vi "Highlight failed parts(Table).vi"(8 "error in (no error)":errorcluster, 10 "Tbl Refnum":refnum<vi>, 11 "Fail array":bool[](array[boolean])) -> (0 "error out":errorcluster)   [LabVIEW 2015, in "ZenGage v3.0 UI.lvclass"]
uses:
  ZenGage v3.0 UI.lvclass
  <vilib>/Utility/miscctls.llb/LVRowAndColumnTypeDef.ctl
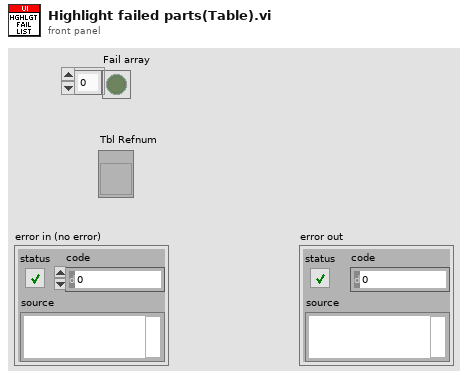
[diagram p1: front panel]
types:
  T1 = typedef "LVRowAndColumnTypeDef.ctl" = cluster{"Row":i32, "Column":i32}
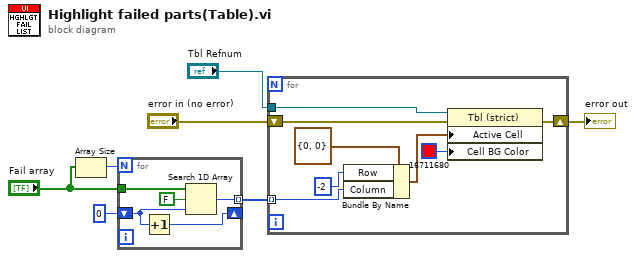
[diagram p0: block diagram]
diagram:
  n1 = Array Size(array="Fail array") -> (size(s)=w3:i32)
  n2 = for {
    N: w3 -> [_]
    tunnel: "Fail array" -> [w12]
    shift-right: [w8] -> _
    shift-left: 0 ("index of element") -> [w9]
    tunnel: [w10] -> w6 mode=indexing
    n3 = Increment(x=w9) -> (x+1=w8:i32)
    n4 = Search 1D Array(1D array=w12, element=FALSE, start index (0)=w9) -> (index of element=w10:i32)
  }
  n5 = for {
    tunnel: w6 -> [w17] mode=indexing
    shift-right: [w15] -> w4
    shift-left: "error in (no error)" -> [w16]
    tunnel: "Tbl Refnum" -> [w13]
    n6 = Bundle By Name(cluster=T1 {"Row"=0, "Column"=0} ("Active Cell:Active Cell"), "Row"=-2, "Column"=w17) -> (w19:T1)
    n7 = property class="Tbl (strict)"(reference=w13, error in=w16, "Active Cell"=w19, "Cell BG Color"=u32 16711680) -> (error out=w15:errorcluster)  [unwired: 1 out]
  }
  "error out" <- w4
